vi "New Verify as Parameterized.vi"(8 "error in":errorcluster, 11 "TestCase in":refnum<class "TestCase.lvclass">) -> (0 "error out":errorcluster, 3 "TestCase out":refnum<class "TestCase.lvclass">)   [LabVIEW 2025, in "VITester.Extension.lvlib"]
uses:
  VITester.Extension.lvlib
  <vilib>/Addons/_JKI Toolkits/VI Tester/TestCase.llb/TestCase.lvclass
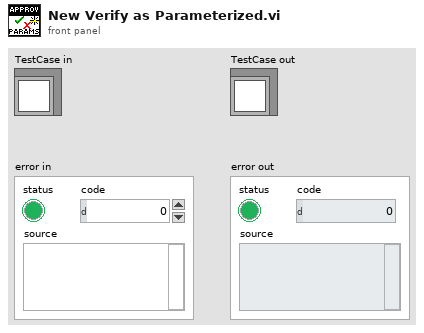
[diagram p1: front panel]
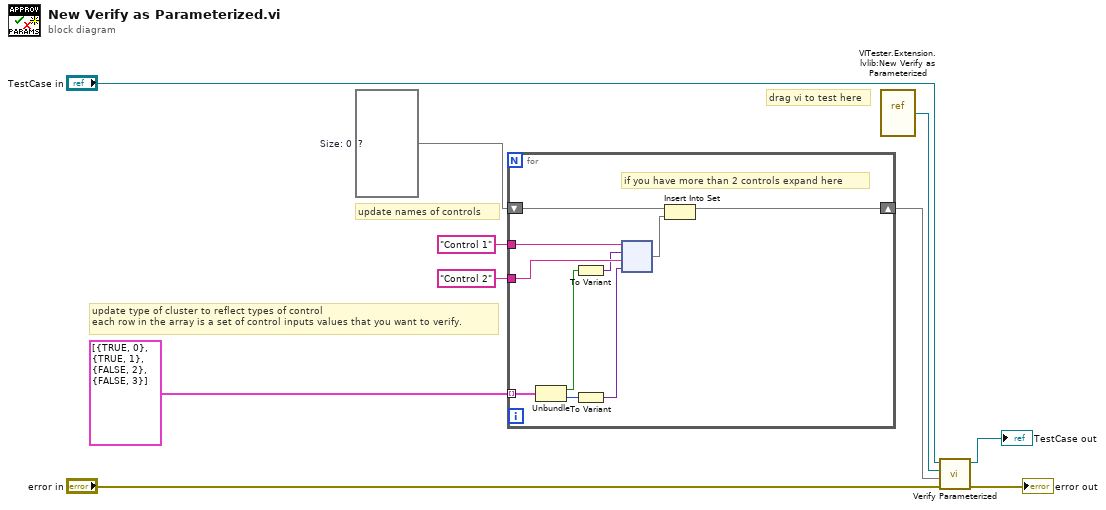
[diagram p0: block diagram]
diagram:
  w4 = set{map{string, variant}} {}  # Size: 0
  # "update type of cluster to reflect types of control\neach row in the array is a set of control inputs values that you want to verify."
  # "update names of controls"
  # "drag vi to test here"
  n1 = for {
    tunnel: "Control 1" -> [w20]
    tunnel: cluster{bool, i32}[] [{TRUE, 0}, {TRUE, 1}, {FALSE, 2}, {FALSE, 3}] -> [w18] mode=indexing
    tunnel: "Control 2" -> [w19]
    shift-right: [w12] -> w3
    shift-left: w4 -> [w11]
    # "if you have more than 2 controls expand here"
    n2 = Unbundle(w18) -> (w17:bool, w16:i32)
    n3 = To Variant(anything=w17) -> (Variant=w14:variant)
    n4 = To Variant(anything=w16) -> (Variant=w13:variant)
    n5 = node(w20, w14, w19, w13) -> (w15:map{string, variant})
    n6 = Insert Into Set(10:w15, 11:w11) -> (3:w12:set{map{string, variant}})  [unwired: 1 out]
  }
  n7 = vi-ref "VITester.Extension.lvlib:New Verify as Parameterized.vi"() -> (w8:refnum<vi>)
  n8 = call "Verify Parameterized.vi"("error in"="error in", "Set of ctl label -> value var"=w3, "VI in"=w8, "TestCase in"="TestCase in") -> ("error out"=→"error out":errorcluster, "TestCase out"=→"TestCase out":refnum<class "TestCase.lvclass">)  [unwired: 6 in]
